vi "VI Tree.vi"   [LabVIEW 2019, in "Pendulum CNT90.lvlib"]
doc: "This is the instrument Driver for Pendulum CNT90, CNT-90XL, CNT-91 Time & Frequency Counter and also supports Fluke PM 6690 timer-counter-analyzer. The VI Tree displays all the user-callable VIs of the instrument driver in an organized table."
uses:
  Pendulum CNT90.lvlib
  Data/Read Measurement (Single).vi
  Data/Low Level/Fetch Measurement (Single).vi
panel:
  # "(c) 2007 National Instruments.  ALL RIGHTS RESERVED."
  # "SEE DIAGRAM\nFOR VI TREE."
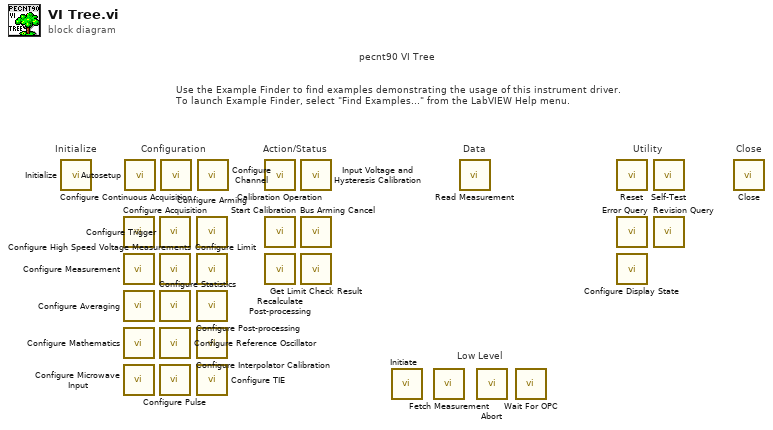
[diagram p0: block diagram]
diagram:
  # "Low Level"
  # "Action/Status"
  # "pecnt90 VI Tree"
  # "Use the Example Finder to find examples demonstrating the usage of this instrument driver.\nTo launch Example Finder, select \"Find Examples...\" from the LabVIEW Help menu."
  # "Configuration"
  # "Utility"
  # "Data"
  # "Close"
  # "Initialize"
  n1 = call "Initialize.vi"() -> ()  [unwired: 10 in, 2 out]
  n2 = call "Configure Acquisition.vi"() -> ()  [unwired: 10 in, 2 out]
  n3 = call "Configure Measurement.vi"() -> ()  [unwired: 14 in, 2 out]
  n4 = call "Configure Averaging.vi"() -> ()  [unwired: 10 in, 2 out]
  n5 = call "Configure Mathematics.vi"() -> ()  [unwired: 14 in, 2 out]
  n6 = call "Configure Microwave Input.vi"() -> ()  [unwired: 10 in, 2 out]
  n7 = call "Autosetup.vi"() -> ()  [unwired: 10 in, 2 out]
  n8 = call "Configure Trigger.vi"() -> ()  [unwired: 10 in, 2 out]
  n9 = call "Configure High Speed Voltage Measurements.vi"() -> ()  [unwired: 10 in, 2 out]
  n10 = call "Configure Statistics.vi"() -> ()  [unwired: 10 in, 2 out]
  n11 = call "Configure Reference Oscillator.vi"() -> ()  [unwired: 10 in, 2 out]
  n12 = call "Configure Pulse.vi"() -> ()  [unwired: 14 in, 2 out]
  n13 = call "Configure Continuous Acquisition.vi"() -> ()  [unwired: 10 in, 2 out]
  n14 = call "Configure Arming.vi"() -> ()  [unwired: 14 in, 2 out]
  n15 = call "Configure Limit.vi"() -> ()  [unwired: 10 in, 2 out]
  n16 = call "Configure Post-processing.vi"() -> ()  [unwired: 10 in, 2 out]
  n17 = call "Configure Interpolator Calibration.vi"() -> ()  [unwired: 10 in, 2 out]
  n18 = call "Configure TIE.vi"() -> ()  [unwired: 10 in, 2 out]
  n19 = call "Configure Channel.vi"() -> ()  [unwired: 14 in, 2 out]
  n20 = call "Calibration Operation.vi"() -> ()  [unwired: 14 in, 2 out]
  n21 = call "Start Calibration.vi"() -> ()  [unwired: 10 in, 2 out]
  n22 = call "Recalculate Post-processing.vi"() -> ()  [unwired: 10 in, 2 out]
  n23 = call "Input Voltage and Hysteresis Calibration.vi"() -> ()  [unwired: 10 in, 2 out]
  n24 = call "Bus Arming Cancel.vi"() -> ()  [unwired: 10 in, 2 out]
  n25 = call "Get Limit Check Result.vi"() -> ()  [unwired: 9 in, 3 out]
  n26 = call "Initiate.vi"() -> ()  [unwired: 10 in, 2 out]
  n27 = call-poly "Fetch Measurement.vi"() -> ()  [unwired: 9 in, 3 out]
  n28 = call-poly "Read Measurement.vi"() -> ()  [unwired: 9 in, 3 out]
  n29 = call "Abort.vi"() -> ()  [unwired: 10 in, 2 out]
  n30 = call "Wait For OPC.vi"() -> ()  [unwired: 9 in, 3 out]
  n31 = call "Reset.vi"() -> ()  [unwired: 10 in, 2 out]
  n32 = call "Error Query.vi"() -> ()  [unwired: 8 in, 4 out]
  n33 = call "Configure Display State.vi"() -> ()  [unwired: 10 in, 2 out]
  n34 = call "Self-Test.vi"() -> ()  [unwired: 8 in, 4 out]
  n35 = call "Revision Query.vi"() -> ()  [unwired: 8 in, 4 out]
  n36 = call "Close.vi"() -> ()  [unwired: 11 in, 1 out]
